vi "Distance Formula.vi"(4 "Point2":cluster{"x":dbl, "y":dbl}, 5 "Point1":cluster{"x":dbl, "y":dbl}) -> (1 "Distance":dbl)   [LabVIEW 2018, in "Pure Pursuit.lvlib"]
uses:
  Pure Pursuit.lvlib
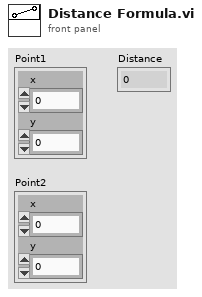
[diagram p1: front panel]
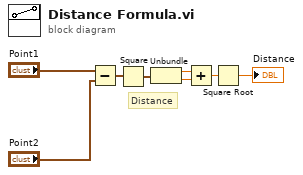
[diagram p0: block diagram]
diagram:
  # "Distance"
  n1 = Subtract(x="Point1", y="Point2") -> (x-y=w7:cluster{"x":dbl, "y":dbl})
  n2 = Square(x=w7) -> (x^2=w8:cluster{"x":dbl, "y":dbl})
  n3 = Unbundle(w8) -> ("x"=w3:dbl, "y"=w4:dbl)
  n4 = Add(x=w3, y=w4) -> (x+y=w5:dbl)
  n5 = Square Root(x=w5) -> (sqrt(x)=→"Distance":dbl)
